vi "5492_ButtonDebounced.vi"(0 "Button":bool, 1 "Last Pressed":dbl, 2 "Current":dbl) -> (5 "Button Debounced":bool, 6 "Last Pressed Out":dbl)   [LabVIEW 2017]
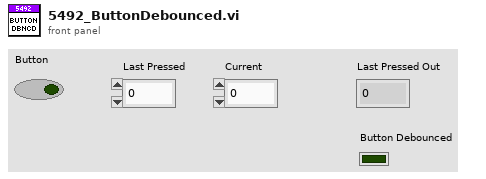
[diagram p1: front panel]
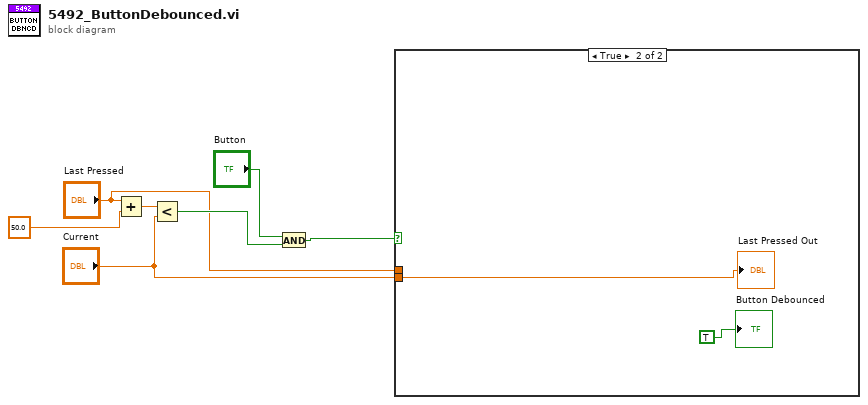
[diagram p0: block diagram]
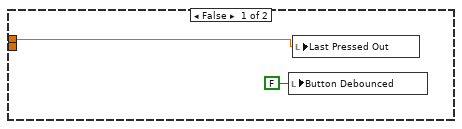
[diagram p2: hidden frame]
diagram:
  n1 = Add(x="Last Pressed", y=50.0 ("Current")) -> (x+y=w6:dbl)
  n2 = Less?(x=w6, y="Current") -> (x < y?=w4:bool)
  n3 = And(x="Button", y=w4) -> (x .and. y?=w3:bool)
  n4 = case shown="True" w3 {
    tunnel: "Last Pressed" -> [w8 _]
    tunnel: "Current" -> [_ w10]
    frame False {
      n5 = local write "Button Debounced"(FALSE ("Button Debounced")) -> ()
      n6 = local write "Last Pressed Out"(w8) -> ()
    }
    frame True {
      "Last Pressed Out" <- w10
      "Button Debounced" <- TRUE ("Button Debounced")
    }
  }
